vi "Module Type.vi"(11 "TestModule in":refnum<class "TestModule.lvclass">) -> (2 "Module Type":string)   [LabVIEW 2020, in "VolatusScratch.lvlib" / "TestModule.lvclass"]
uses:
  TestModule.lvclass
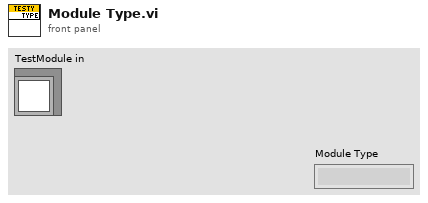
[diagram p1: front panel]
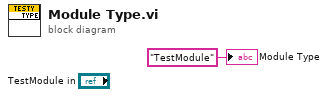
[diagram p0: block diagram]
diagram:
  "Module Type" <- "TestModule" ("Module Type")
